vi "Find Parse State Queue from Event Strcture.vi"(8 "error in (no error)":errorcluster, 11 "EvntStruct Refnum":refnum<vi>) -> (0 "error out":errorcluster, 1 "CaseStructure":refnum<vi>, 2 "Parse State Queue":refnum<vi>)   [LabVIEW 2017, in "csmHelper-Relationship.lvlib"]
uses:
  csmHelper-Relationship.lvlib
  CSM-Helper.lvclass
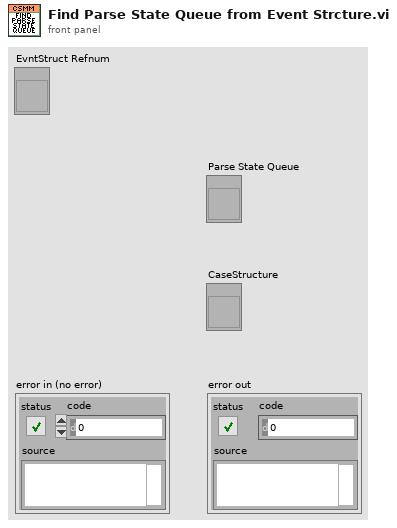
[diagram p1: front panel]
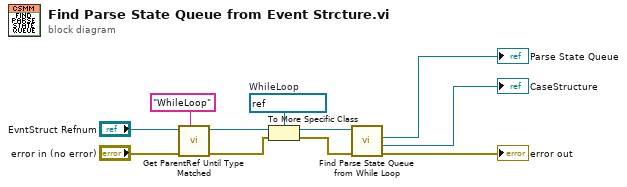
[diagram p0: block diagram]
diagram:
  w7 = refnum<vi> refnum  # WhileLoop
  n1 = call "Get ParentRef Until Type Matched.vi"("Class Name"="WhileLoop", "Error in"="error in (no error)", "reference in"="EvntStruct Refnum") -> ("Error out"=w1:errorcluster, "Target Ref"=w9:refnum<vi>)  [unwired: 5 in]
  n2 = To More Specific Class(target class=w7, reference=w9, error in=w1) -> (specific class reference=w8:refnum<vi>, error out=w6:errorcluster)
  n3 = call "Find Parse State Queue from While Loop.vi"("error in (no error)"=w6, "WhileLoop in"=w8) -> ("error out"=→"error out":errorcluster, "CaseStructure"=→"CaseStructure":refnum<vi>, "Parse State Queue"=→"Parse State Queue":refnum<vi>)  [unwired: 6 in, 1 out]
